vi "edit_data (SubVI).vi"(10 "data in":string) -> (0 "error bool out":bool, 1 "Enum":T1, 2 "data out":string)   [LabVIEW 2015]
uses:
  enum_typedef.ctl
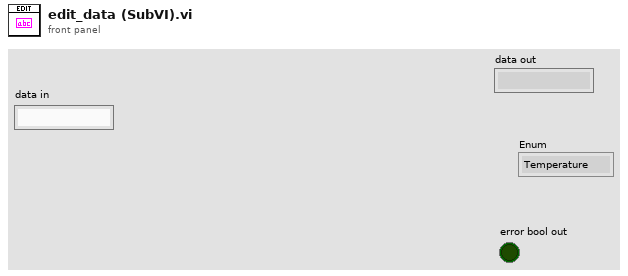
[diagram p1: front panel]
types:
  T1 = typedef "enum_typedef.ctl" = enum16{"Temperature", "X axis", "Y axis", "Z axis"}
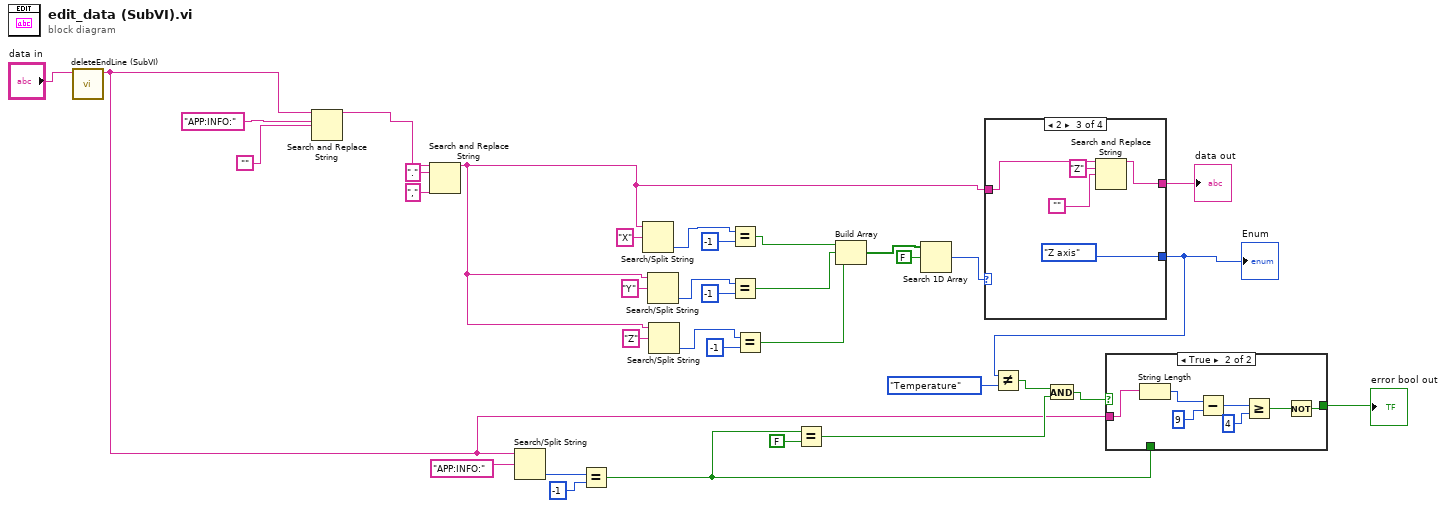
[diagram p0: block diagram]
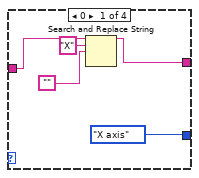
[diagram p3: hidden frame]
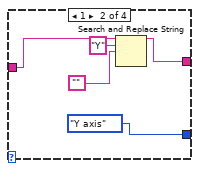
[diagram p4: hidden frame]
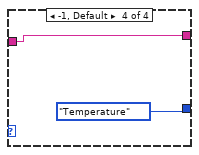
[diagram p5: hidden frame]
diagram:
  n1 = call "deleteEndLine (SubVI).vi"("read buffer"="data in") -> ("result string"=w1:string)  [unwired: 10 in]
  n2 = Search and Replace String(input string=w1, search string="APP:INFO:", replace string="") -> (result string=w30:string)  [unwired: 5 in, 3 out]
  n3 = Search and Replace String(input string=w30, search string=".", replace string="," ("replace string (\"\")")) -> (result string=w14:string)  [unwired: 5 in, 3 out]
  n4 = Search/Split String(string=w1, search string/char (-)="APP:INFO:") -> (offset of match=w11:i32)  [unwired: 1 in, 2 out]
  n5 = Equal?(x=w11, y=-1) -> (x = y?=w3:bool)
  n6 = Search/Split String(string=w14, search string/char (-)="X") -> (offset of match=w22:i32)  [unwired: 1 in, 2 out]
  n7 = Search/Split String(string=w14, search string/char (-)="Y") -> (offset of match=w21:i32)  [unwired: 1 in, 2 out]
  n8 = Search/Split String(string=w14, search string/char (-)="Z") -> (offset of match=w23:i32)  [unwired: 1 in, 2 out]
  n9 = Equal?(x=w22, y=-1) -> (x = y?=w20:bool)
  n10 = Equal?(x=w21, y=-1) -> (x = y?=w19:bool)
  n11 = Equal?(x=w23, y=-1) -> (x = y?=w18:bool)
  n12 = Equal?(x=w3, y=FALSE) -> (x = y?=w5:bool)
  n13 = Build Array(w20, w19, w18) -> (w17:bool[])
  n14 = Search 1D Array(1D array=w17, element=FALSE) -> (index of element=w15:i32)  [unwired: 1 in]
  n15 = case shown="2" w15 {
    tunnel: [enum_typedef."X axis" ("Enum 2") enum_typedef."Y axis" ("Enum 2") enum_typedef."Z axis" ("Enum 2") enum_typedef."Temperature" ("Enum 2")] -> w8
    tunnel: w14 -> [w40 w43 w48 w52]
    tunnel: [w39 w42 w47 w52] -> w13
    frame 0 {
      n16 = Search and Replace String(input string=w40, search string="X", replace string="") -> (result string=w39:string)  [unwired: 5 in, 3 out]
    }
    frame 1 {
      n17 = Search and Replace String(input string=w43, search string="Y", replace string="") -> (result string=w42:string)  [unwired: 5 in, 3 out]
    }
    frame 2 {
      n18 = Search and Replace String(input string=w48, search string="Z", replace string="") -> (result string=w47:string)  [unwired: 5 in, 3 out]
    }
    frame -1, Default {
    }
  }
  "data out" <- w13
  "Enum" <- w8
  n19 = Not Equal?(x=w8, y=enum_typedef."Temperature") -> (x != y?=w6:bool)
  n20 = And(x=w6, y=w5) -> (x .and. y?=w4:bool)
  n21 = case shown="True" w4 {
    tunnel: w3 -> [w53 _]
    tunnel: [w53 w54] -> w2
    tunnel: w1 -> [_ w60]
    frame False {
    }
    frame True {
      n22 = String Length(string=w60) -> (length=w59:i32)
      n23 = Subtract(x=w59, y=9) -> (x-y=w57:i32)
      n24 = Greater Or Equal?(x=w57, y=4) -> (x >= y?=w55:bool)
      n25 = Not(x=w55) -> (.not. x?=w54:bool)
    }
  }
  "error bool out" <- w2
